vi "Get Tables.vi"(8 "error in (no error)":errorcluster, 11 "Data.PG":refnum<class "Data.PGSQL.lvclass">) -> (0 "error out":errorcluster, 1 "Table Paths":string[](array[string]), 2 "Table Names":string[](array[string]), 3 "Data.PG out":refnum<class "Data.PGSQL.lvclass">)   [LabVIEW 2013, in "Data.PGSQL.lvclass"]
uses:
  Data.PGSQL.lvclass
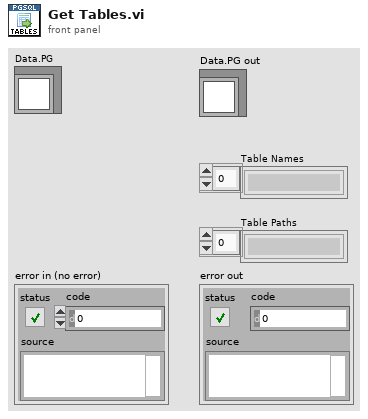
[diagram p1: front panel]
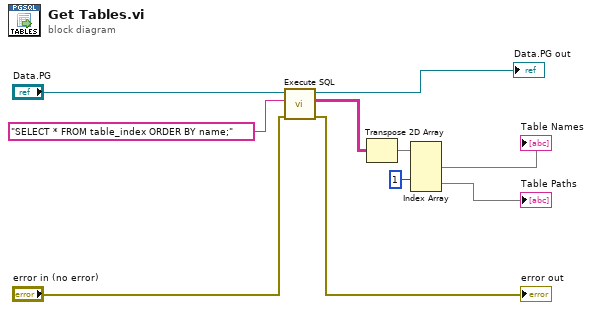
[diagram p0: block diagram]
diagram:
  n1 = call "Execute SQL.vi"("error in"="error in (no error)", "SQL"="SELECT * FROM table_index ORDER BY name;" ("command"), "Data.PG"="Data.PG") -> ("error out"=→"error out":errorcluster, "Result"=w3:string[][], "Data.PG out"=→"Data.PG out":refnum<class "Data.PGSQL.lvclass">)  [unwired: 6 in]
  n2 = Transpose 2D Array(2D array=w3) -> (transposed array=w6:string[][])
  n3 = Index Array(array=w6, index (row) #2=1 ("index (row)")) -> (element #1=→"Table Names":string[], element #2=→"Table Paths":string[])  [unwired: 3 in]
